vi "Disable steppers.vi"(8 "error in (no error)":errorcluster, 11 "VISA resource name":refnum<visa-resource-name>) -> (0 "error out":errorcluster, 3 "VISA resource name out":refnum<visa-resource-name>)   [LabVIEW 2023, in "Marlin Instrument Driver.lvlib"]
doc: "Returns the current state of the configured X, Y, Z endstops. Takes into account any 'inverted endstop' settings, so one can confirm that the machine is interpreting the endstops correctly."
uses:
  Marlin Instrument Driver.lvlib
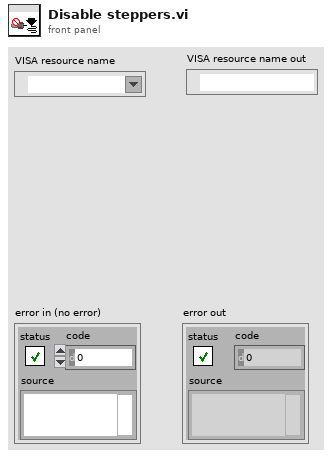
[diagram p1: front panel]
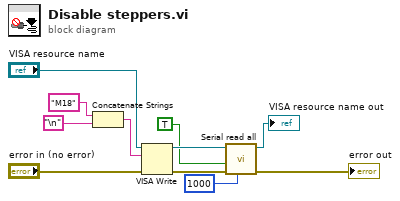
[diagram p0: block diagram]
diagram:
  n1 = Concatenate Strings("M18" ("command"), "\n") -> (w8:string)
  n2 = VISA Write(VISA resource name="VISA resource name", write buffer=w8, error in (no error)="error in (no error)") -> (VISA resource name out=w6:refnum<visa-resource-name>, error out=w7:errorcluster)  [unwired: 1 out]
  n3 = call "Serial read all.vi"("timeout (10000ms)"=u32 1000, "error in (no error)"=w7, "Wait for OK"=TRUE, "VISA Refnum in"=w6) -> ("error out"=→"error out":errorcluster, "VISA Refnum out"=→"VISA resource name out":refnum<visa-resource-name>)  [unwired: 4 in, 2 out]
